vi "Read All Data.vi"(4 "Error In":errorcluster, 7 "Instance Name":T1) -> (0 "Error Out":errorcluster, 3 "TC Data":T2(array[cluster]))   [LabVIEW 2015, in "Temperature Controller Data Buffer.lvlib"]
uses:
  Temperature Controller Data Buffer.lvlib
  _libraries/Startup Processes/_typedefs/Subpanel Names.ctl
  _libraries/Startup Processes/Startup Processes.lvlib
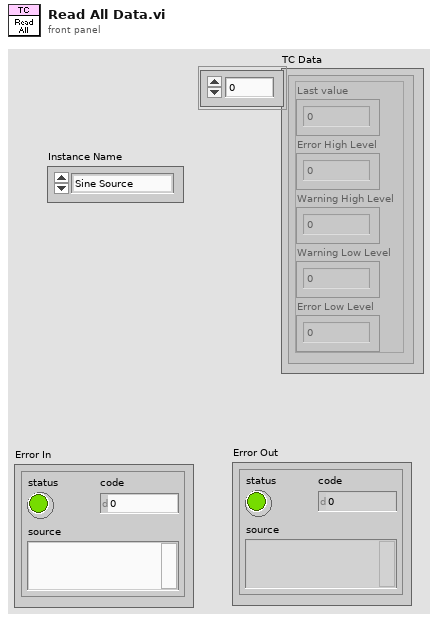
[diagram p1: front panel]
types:
  T1 = typedef "Startup Processes.lvlib/Subpanel Names.ctl" = enum16{"Sine Source", "Ramp Source", "Hen House TC", "Dog House TC", "Out House TC"}
  T2 = cluster{"Last value":dbl, "Error High Level":dbl, "Warning High Level":dbl, "Warning Low Level":dbl, "Error Low Level":dbl}[]
  T3 = typedef "Temperature Controller Data Buffer.lvlib/buffer data typedef.ctl" = cluster{"TC Data":cluster{"Last value":dbl, "Error High Level":dbl, "Warning High Level":dbl, "Warning Low Level":dbl, "Error Low Level":dbl}[], "Counter":i32}
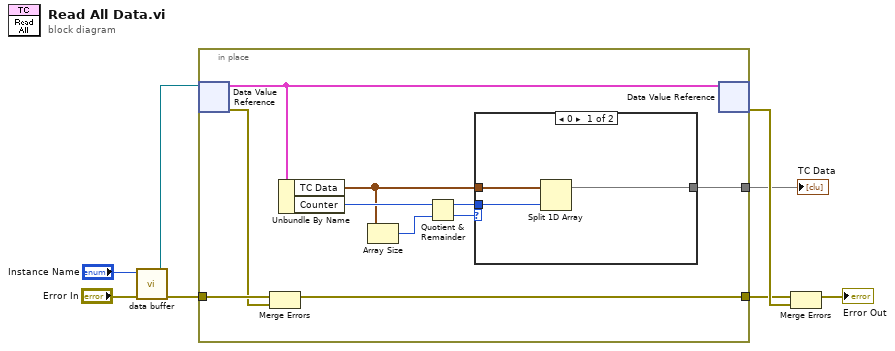
[diagram p0: block diagram]
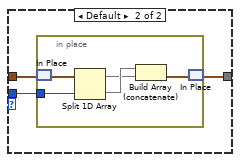
[diagram p2: hidden frame]
diagram:
  n1 = call "data buffer.vi"("Error In"="Error In", "Instance Name"="Instance Name") -> ("Error Out"=w3:errorcluster, "DVR"=w7:refnum<data-value>)  [unwired: 4 in]
  n2 = in-place {
    in-place-border: [w17] -> w4
    in-place-border: w3 -> [w16]
    in-place-border: [w14] -> w2
    n3 = in-place-dvr #1(w7) -> (w18:T3, w15:errorcluster)
    n4 = Merge Errors(w16, w15) -> (w14:errorcluster)
    n5 = Unbundle By Name(w18) -> ("TC Data"=w10:T2, "Counter"=w13:i32)
    n6 = Array Size(array=w10) -> (size(s)=w9:i32)
    n7 = Quotient & Remainder(x=w13, y=w9) -> (x-y*floor(x/y)=w11:i32, floor(x/y)=w12:i32)
    n8 = case shown="0" w12 {
      tunnel: w10 -> [w21 w24]
      tunnel: [w19 w23] -> w17
      tunnel: w11 -> [w20 w22]
      frame 0 {
        n9 = Split 1D Array(array=w21, index=w20) -> (first subarray=w19:T2)  [unwired: 1 out]
      }
      frame Default {
        n10 = in-place {
          in-place-border: w22 -> [w29]
          n11 = in-place-match #2(w24) -> (w26:T2)
          n12 = Split 1D Array(array=w26, index=w29) -> (first subarray=w27:T2, second subarray=w28:T2)
          n13 = Build Array (concatenate)(w28, w27) -> (w25:T2)
          n14 = in-place-match #2(w25) -> (w23:T2)
        }
      }
    }
    n15 = in-place-dvr #1(w18) -> (w8:errorcluster)  [unwired: 1 out]
  }
  "TC Data" <- w4
  n16 = Merge Errors(w2, w8) -> (→"Error Out":errorcluster)
